vi "Subscribe (SingleTopic).vi"(6 "timeout (100ms)":i32=100, 8 "error in (no error)":errorcluster, 9 "QoS":T1, 10 "Topic Filter":string, 11 "MQTT_Base in":refnum<class "MQTT_Base.lvclass">) -> (0 "error out":errorcluster, 1 "Ack":bool, 3 "MQTT_Base out":refnum<class "MQTT_Base.lvclass">)   [LabVIEW 2013, in "MQTT Base.lvlib" / "MQTT_Base.lvclass"]
uses:
  MQTT_Base.lvclass
  <vilib>/LabVIEW Open Source Project/MQTT Control Packets/Control Packets/ControlPacket/QualityOfService -- enum.ctl
  <vilib>/LabVIEW Open Source Project/MQTT Control Packets/Control Packets/SUBSCRIBE/Topic Subscription -- cluster.ctl
  <vilib>/LabVIEW Open Source Project/MQTT Control Packets/Control Packets/SUBSCRIBE/SUBSCRIBE.lvclass
  <vilib>/LabVIEW Open Source Project/MQTT Control Packets/Control Packets/ControlPacket/ControlPacket.lvclass
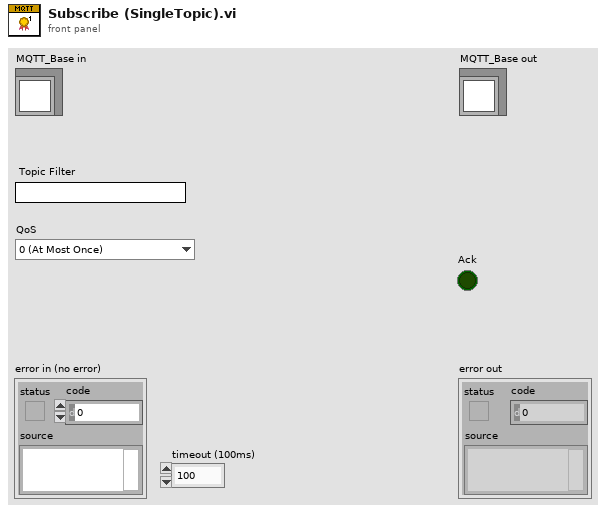
[diagram p1: front panel]
types:
  T1 = typedef "MQTT_Control_Packets.lvlib/ControlPacket.lvclass/QualityOfService -- enum.ctl" = enum16{"0 (At Most Once)", "1 (At Least Once)", "2 (Exactly Once)"}
  T2 = typedef "MQTT_Control_Packets.lvlib/SUBSCRIBE.lvclass/Topic Subscription -- cluster.ctl" = cluster{"Topic Filter":string, "QoS":T1}
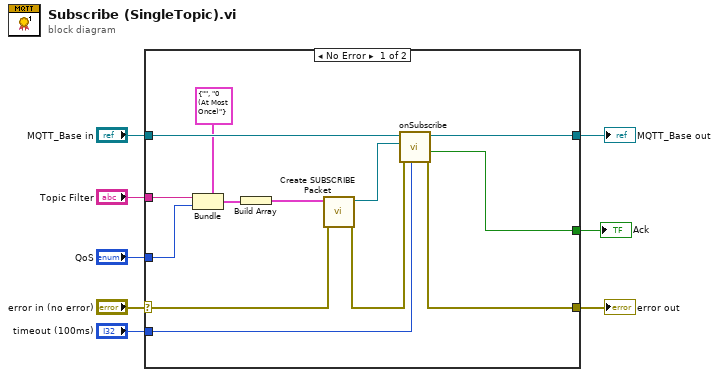
[diagram p0: block diagram]
diagram:
  n1 = case shown="No Error" "error in (no error)" {
    selector: "error in (no error)" -> [w16 w23]
    tunnel: [w19 w23] -> w7
    tunnel: [w20 w22] -> w5
    tunnel: "MQTT_Base in" -> [w21 w22]
    tunnel: "Topic Filter" -> [w15 _]
    tunnel: "QoS" -> [w14 _]
    tunnel: "timeout (100ms)" -> [w10 _]
    tunnel: [w9 _] -> w1
    frame No Error {
      n2 = Bundle(cluster=T2 {"Topic Filter"="", "QoS"=enum."0 (At Most Once)"} ("Topic Subscription"), "Topic Filter"=w15, "QoS"=w14) -> (w13:T2)
      n3 = Build Array(w13) -> (w12:T2[])
      n4 = call <vilib>:"Create SUBSCRIBE Packet.vi"("error in (no error)"=w16, "Topic Subscriptions"=w12) -> ("error out"=w17:errorcluster, "SUBSCRIBE out"=w18:refnum<class "SUBSCRIBE.lvclass">)  [unwired: 7 in, 1 out]
      n5 = call-dynamic "onSubscribe.vi"("timeout (100ms)"=w10, "error in (no error)"=w17, "SUBSCRIBE"=w18, "MQTT_Base in"=w21) -> ("error out"=w19:errorcluster, "Ack?"=w9:bool, "MQTT_Base out"=w20:refnum<class "MQTT_Base.lvclass">)  [unwired: 4 in, 1 out]
    }
    frame Error {
    }
  }
  "error out" <- w7
  "MQTT_Base out" <- w5
  "Ack" <- w1
